vi "ClientUtilities3.vi"(1 "Action":enum16{"Open Connection"}(ring), 2 "ServerPort":u16=2402, 3 "ServerName":string="tester") -> (0 "Error":bool)   [LabVIEW 2014]
uses:
  EngineeringGlobals.vi
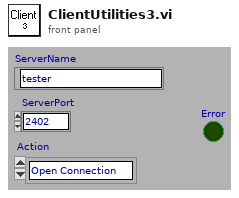
[diagram p1: front panel]
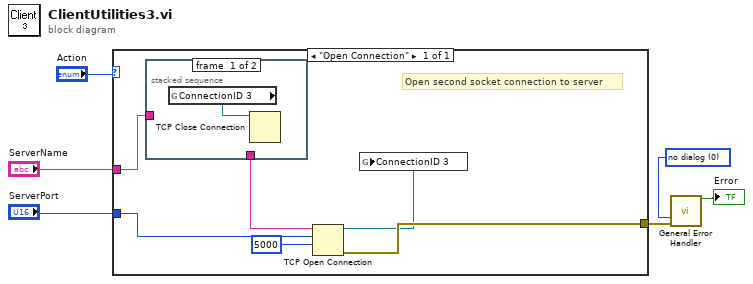
[diagram p0: block diagram]
diagram:
  w3 = u16 0 items=["no dialog", "OK message", "continue or stop message"] ("type of dialog (OK msg:1)")
  n1 = case shown="\"Open Connection\"" "Action" {
    tunnel: [w11] -> w5
    tunnel: "ServerName" -> [w9]
    tunnel: "ServerPort" -> [w12]
    frame "Open Connection" {
      # "Open second socket connection to server"
      n2 = stacked-sequence {
        tunnel: w9 -> [_ w14]
        tunnel: [_ w14] -> w8
        frame #0 {
          n3 = global read "EngineeringGlobals.vi" "ConnectionID 3"() -> (w13:refnum<k5>)
          n4 = TCP Close Connection(connection ID=w13) -> ()  [unwired: 2 in, 2 out]
        }
        frame #1 {
        }
      }
      n5 = TCP Open Connection(address=w8, remote port or service name=w12, timeout ms (60000)=5000) -> (connection ID=w7:refnum<k5>, error out=w11:errorcluster)  [unwired: 2 in]
      n6 = global write "EngineeringGlobals.vi" "ConnectionID 3"(w7) -> ()
    }
  }
  n7 = call <vilib>:"General Error Handler.vi"("type of dialog (OK msg:1)"=w3, "error in (no error)"=w5) -> ("error?"=→"Error":bool)  [unwired: 9 in, 4 out]
